vi "p1230 open.vi"(8 "error in (no error)":errorcluster, 11 "board_id":u32) -> (0 "error out":errorcluster, 3 "function return":u32)   [LabVIEW 2014]
doc: "unsigned int __stdcall p1230_open(unsigned int board_id);"
uses:
  PCI1230UTIL.dll
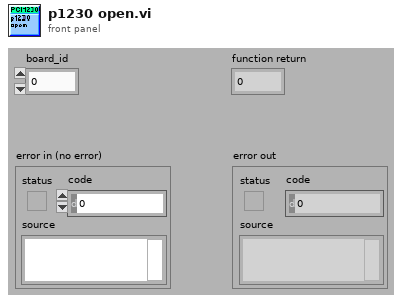
[diagram p1: front panel]
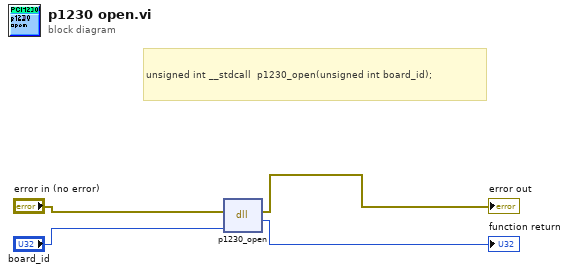
[diagram p0: block diagram]
diagram:
  # "unsigned int __stdcall  p1230_open(unsigned int board_id);"
  n1 = dll-call lib="C:/Users/AICTER/Desktop/PCI-1230/PCI1230_VIs/PCI1230UTIL.dll" fn="p1230_open"(error in="error in (no error)", "board_id"="board_id") -> (error out=→"error out":errorcluster, "return type"=→"function return":u32)  [unwired: 3 in, 1 out]
